vi "Actor Core.vi"(8 "error in":errorcluster, 11 "AE75TX in":refnum<class "AE75TX.lvclass">) -> (0 "error out":errorcluster, 3 "Actor out":refnum<class "Actor.lvclass">)   [LabVIEW 2015, in "AE75TX Actor.lvlib" / "AE75TX.lvclass"]
doc: "(<B>Filename</B>: Actor Framework.lvlib:Actor.lvclass:Actor Core.vi)\n\nReceives messages to the actor, reacts to them, and initiates any error handling that may shut the actor down.\n\nDescendant classes may override this VI to append parallel tasks for the actor to complete while it handles messages. Overrides use the Call Parent Method node."
uses:
  AE75TX.lvclass
  <vilib>/ActorFramework/Actor/Actor.lvclass
  Controls/PV State Selector.ctl
  AE75TX.lvclass/AE75TX.ctl
  Controls/PV Standard Value Cluster.ctl
  Controls/PV Full Data Cluster.ctl
  <vilib>/Modbus/master/Create Master Instance (TCP).vi
  <vilib>/Modbus/slave/Create Slave Instance (TCP).vi
  <vilib>/Modbus/slave/Modbus Slave.lvclass
  <vilib>/Modbus/master/Modbus Master.lvclass
panel:
  out "Deactivate":bool
  out "Activate":bool
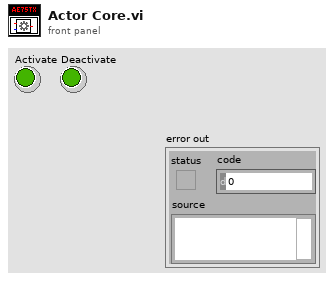
[diagram p1: front panel]
types:
  T1 = typedef "AE75TX Actor.lvlib/AE75TX.lvclass/PV State Selector.ctl" = enum16{"Init", "Read", "Error Check", "Close"}
  T2 = typedef "AE75TX Actor.lvlib/AE75TX.lvclass/PV Full Data Cluster.ctl" = cluster{"PV Standard Values":T3, "Reactive Power (kVAR)":sgl}
  T3 = typedef "AE75TX Actor.lvlib/AE75TX.lvclass/PV Standard Value Cluster.ctl" = cluster{"Va (V)":sgl, "Vb (V)":sgl, "Vc (V)":sgl, "Ia (A)":sgl, "Ib (A)":sgl, "Ic (A)":sgl, "Vdc (V)":sgl, "Idc (A)":sgl, "Frequency (Hz)":sgl, "Line Power (kW)":sgl, "Total Power (kWh)":u32, "PV Input (V)":sgl, "DC Power (kW)":sgl}
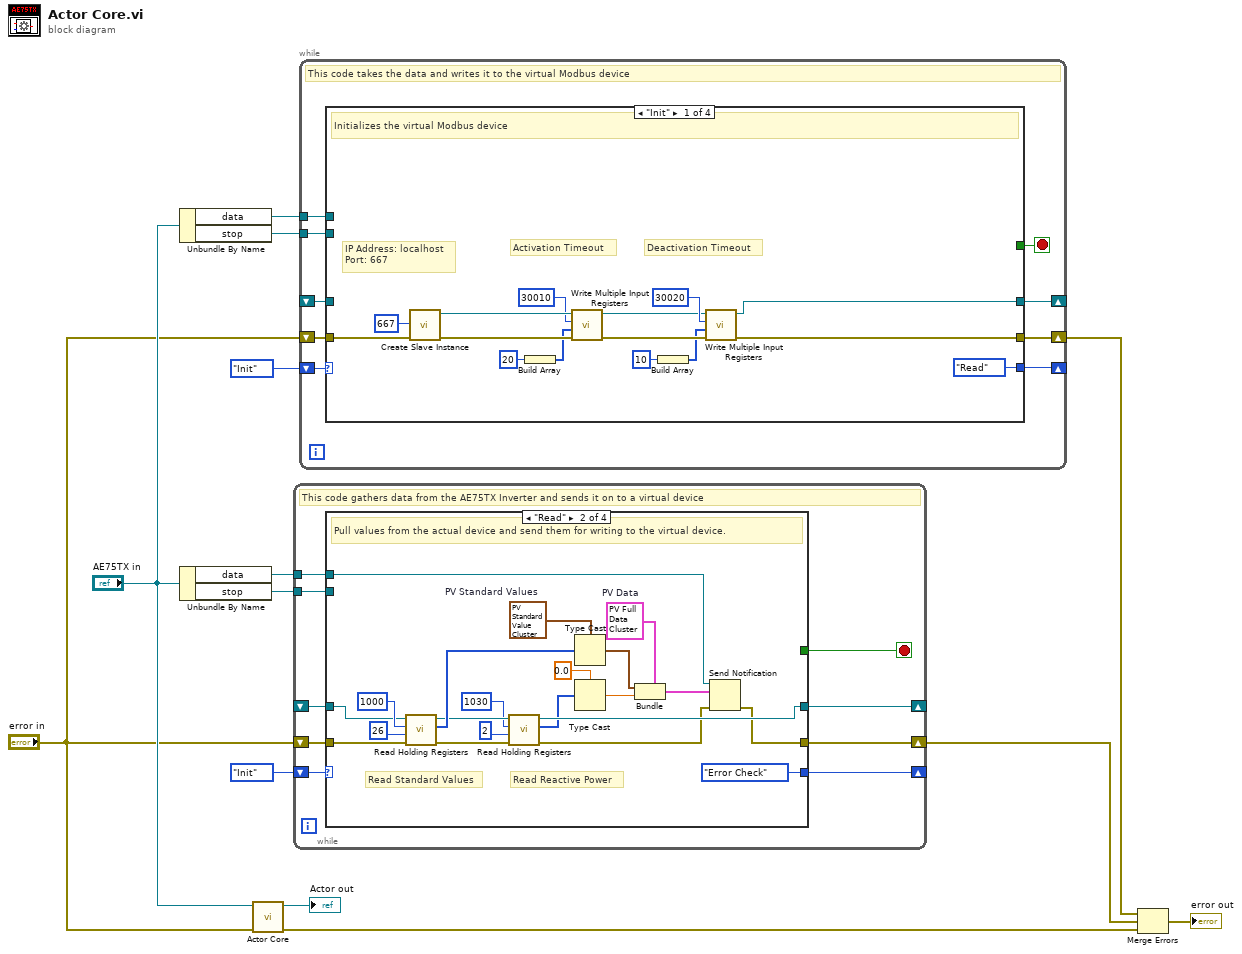
[diagram p0: block diagram]
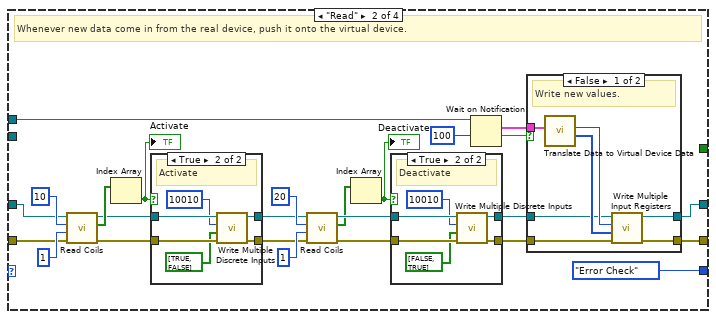
[diagram p2: hidden frame]
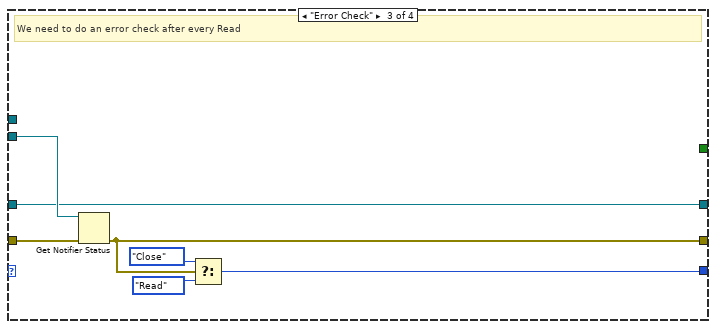
[diagram p6: hidden frame]
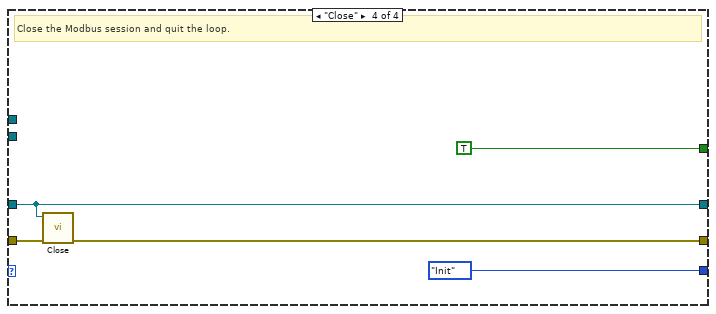
[diagram p7: hidden frame]
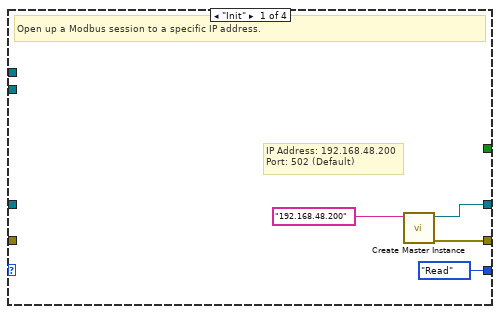
[diagram p8: hidden frame]
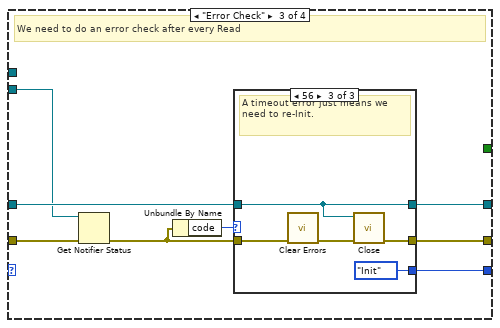
[diagram p9: hidden frame]
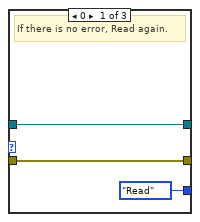
[diagram p10: hidden frame]
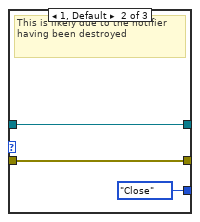
[diagram p11: hidden frame]
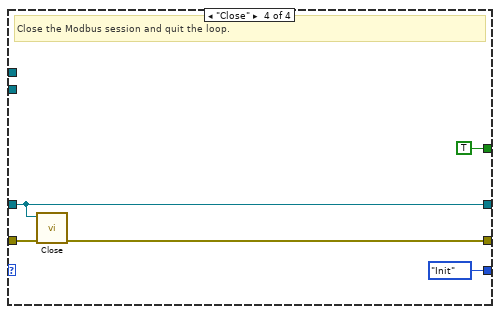
[diagram p12: hidden frame]
diagram:
  n1 = Unbundle By Name("AE75TX in") -> ("data"=w3:refnum<notifier>, "stop"=w2:refnum<notifier>)
  n2 = Unbundle By Name("AE75TX in") -> ("data"=w10:refnum<notifier>, "stop"=w9:refnum<notifier>)
  n3 = call-parent "Actor Core.vi"("error in"="error in", "Actor in"="AE75TX in") -> ("error out"=w13:errorcluster, "Actor out"=→"Actor out":refnum<class "Actor.lvclass">)  [unwired: 8 in]
  n4 = while {
    shift-right: [w20] -> _
    shift-left: PV_State_Selector."Init" -> [w22]
    shift-right: [w21] -> _
    shift-left: _ -> [w19]
    shift-right: [w17] -> w7
    shift-left: "error in" -> [w18]
    tunnel: w10 -> [w16]
    tunnel: w9 -> [w14]
    stop <- w15 stop-if-true
    # "This code gathers data from the AE75TX Inverter and sends it on to a virtual device"
    n5 = case shown="\"Read\"" w22 {
      tunnel: [w25 w37 w51 w68] -> w21
      tunnel: [w24 w27 w54 w70] -> w17
      tunnel: [PV_State_Selector."Read" PV_State_Selector."Error Check" w52 PV_State_Selector."Init"] -> w20
      tunnel: w19 -> [_ w43 w53 w68]
      tunnel: w18 -> [_ w42 w50 w71]
      tunnel: [_ _ _ TRUE ("stop")] -> w15
      tunnel: w16 -> [_ w30 _ _]
      tunnel: w14 -> [_ _ w48 _]
      frame "Init" {
        # "IP Address: 192.168.48.200\nPort: 502 (Default)"
        # "Open up a Modbus session to a specific IP address."
        n6 = call-poly <vilib>:"Create Master Instance.vi"("address"="192.168.48.200") -> ("error out"=w24:errorcluster, "TCP master instance"=w25:refnum<class "Modbus Master.lvclass">)  [unwired: 9 in]
      }
      frame "Read" {
        w31 = T2 {"PV Standard Values"={"Va (V)"=0.0, "Vb (V)"=0.0, "Vc (V)"=0.0, "Ia (A)"=0.0, "Ib (A)"=0.0, "Ic (A)"=0.0, "Vdc (V)"=0.0, "Idc (A)"=0.0, "Frequency (Hz)"=0.0, "Line Power (kW)"=0.0, "Total Power (kWh)"=0, "PV Input (V)"=0.0, "DC Power (kW)"=0.0}, "Reactive Power (kVAR)"=0.0}  # PV Data
        w46 = T3 {"Va (V)"=0.0, "Vb (V)"=0.0, "Vc (V)"=0.0, "Ia (A)"=0.0, "Ib (A)"=0.0, "Ic (A)"=0.0, "Vdc (V)"=0.0, "Idc (A)"=0.0, "Frequency (Hz)"=0.0, "Line Power (kW)"=0.0, "Total Power (kWh)"=0, "PV Input (V)"=0.0, "DC Power (kW)"=0.0}  # PV Standard Values
        # "Read Reactive Power"
        # "Read Standard Values"
        # "Pull values from the actual device and send them for writing to the virtual device."
        n7 = call-dynamic "Read Holding Registers.vi"("error in (no error)"=w42, "number of holding registers"=u16 26, "starting address"=u16 1000, "Modbus master in"=w43) -> ("error out"=w39:errorcluster, "register values"=w47:u16[], "Modbus master out"=w40:refnum<class "Modbus Master.lvclass">)  [unwired: 5 in]
        n8 = call-dynamic "Read Holding Registers.vi"("error in (no error)"=w39, "number of holding registers"=u16 2, "starting address"=u16 1030, "Modbus master in"=w40) -> ("error out"=w28:errorcluster, "register values"=w35:u16[], "Modbus master out"=w37:refnum<class "Modbus Master.lvclass">)  [unwired: 5 in]
        n9 = Type Cast(type=w46, x=w47) -> (*(type *) &x=w33:T3)
        n10 = Type Cast(type=sgl 0.0, x=w35) -> (*(type *) &x=w32:sgl)
        n11 = Bundle(cluster=w31, "PV Standard Values"=w33, "Reactive Power (kVAR)"=w32) -> (w29:T2)
        n12 = Send Notification(notification=w29, notifier=w30, error in (no error)=w28) -> (error out=w27:errorcluster)  [unwired: 1 out]
      }
      frame "Error Check" {
        # "We need to do an error check after every Read"
        n13 = Get Notifier Status(notifier=w48, error in (no error)=w50) -> (error out=w49:errorcluster)  [unwired: 4 out]
        n14 = Unbundle By Name(w49) -> ("code"=w55:i32)
        n15 = case shown="56" w55 {
          tunnel: w49 -> [w58 w59 w66]
          tunnel: [w58 w59 w64] -> w54
          tunnel: w53 -> [w57 w60 w62]
          tunnel: [PV_State_Selector."Read" PV_State_Selector."Close" PV_State_Selector."Init"] -> w52
          tunnel: [w57 w60 w62] -> w51
          frame 0 {
            # "If there is no error, Read again."
          }
          frame 1, Default {
            # "This is likely due to the notifier having been destroyed"
          }
          frame 56 {
            # "A timeout error just means we need to re-Init."
            n16 = call <vilib>:"Clear Errors.vi"("error in (no error)"=w66) -> ("error out"=w65:errorcluster)  [unwired: 5 in, 1 out]
            n17 = call-dynamic "Close.vi"("error in (no error)"=w65, "Modbus master in"=w62) -> ("error out"=w64:errorcluster)  [unwired: 9 in]
          }
        }
      }
      frame "Close" {
        # "Close the Modbus session and quit the loop."
        n18 = call-dynamic "Close.vi"("error in (no error)"=w71, "Modbus master in"=w68) -> ("error out"=w70:errorcluster)  [unwired: 9 in]
      }
    }
  }
  n19 = while {
    shift-right: [w80] -> _
    shift-left: _ -> [w76]
    shift-right: [w79] -> w1
    shift-left: "error in" -> [w75]
    tunnel: w3 -> [w74]
    tunnel: w2 -> [w73]
    shift-right: [w72] -> _
    shift-left: PV_State_Selector."Init" -> [w78]
    stop <- w77 stop-if-true
    # "This code takes the data and writes it to the virtual Modbus device"
    n20 = case shown="\"Init\"" w78 {
      tunnel: [w83 w111 w147 w153] -> w80
      tunnel: [w82 w112 w148 w154] -> w79
      tunnel: [PV_State_Selector."Read" PV_State_Selector."Error Check" w149 PV_State_Selector."Init"] -> w72
      tunnel: [_ _ _ TRUE ("stop")] -> w77
      tunnel: w76 -> [_ w110 w147 w153]
      tunnel: w75 -> [w81 w109 w146 w155]
      tunnel: w74 -> [_ w119 _ _]
      tunnel: w73 -> [_ _ w152 _]
      frame "Init" {
        # "Deactivation Timeout"
        # "Activation Timeout"
        # "IP Address: localhost\nPort: 667"
        # "Initializes the virtual Modbus device"
        n21 = call-poly <vilib>:"Create Slave Instance.vi"("error in (no error)"=w81, "port (502)"=u16 667) -> ("error out"=w92:errorcluster, "TCP slave instance"=w93:refnum<class "Modbus Slave.lvclass">)  [unwired: 8 in]
        n22 = Build Array(u16 20 ("Register")) -> (w85:u16[])
        n23 = call-dynamic "Write Multiple Input Registers.vi"("error in (no error)"=w92, "input register values"=w85, "starting address"=u16 30010, "Modbus slave in"=w93) -> ("error out"=w88:errorcluster, "Modbus slave out"=w89:refnum<class "Modbus Slave.lvclass">)  [unwired: 6 in]
        n24 = Build Array(u16 10 ("Register")) -> (w84:u16[])
        n25 = call-dynamic "Write Multiple Input Registers.vi"("error in (no error)"=w88, "input register values"=w84, "starting address"=u16 30020, "Modbus slave in"=w89) -> ("error out"=w82:errorcluster, "Modbus slave out"=w83:refnum<class "Modbus Slave.lvclass">)  [unwired: 6 in]
      }
      frame "Read" {
        # "Whenever new data come in from the real device, push it onto the virtual device."
        n26 = call-dynamic "Read Coils.vi"("error in (no error)"=w109, "number of coils"=u16 1, "starting address"=u16 10, "Modbus slave in"=w110) -> ("error out"=w114:errorcluster, "coil values"=w115:bool[], "Modbus slave out"=w113:refnum<class "Modbus Slave.lvclass">)  [unwired: 5 in]
        n27 = Index Array(array=w115) -> (element=w97:bool)  [unwired: 1 in]
        "Activate" <- w97
        n28 = case shown="True" w97 {
          tunnel: w114 -> [w138 w144]
          tunnel: w113 -> [w139 w145]
          tunnel: [w139 w141] -> w103
          tunnel: [w138 w140] -> w102
          frame False {
          }
          frame True {
            # "Activate"
            n29 = call-dynamic "Write Multiple Discrete Inputs.vi"("error in (no error)"=w144, "discrete input values"=bool[] [TRUE, FALSE], "starting address"=u16 10010, "Modbus slave in"=w145) -> ("error out"=w140:errorcluster, "Modbus slave out"=w141:refnum<class "Modbus Slave.lvclass">)  [unwired: 6 in]
          }
        }
        n30 = call-dynamic "Read Coils.vi"("error in (no error)"=w102, "number of coils"=u16 1, "starting address"=u16 20, "Modbus slave in"=w103) -> ("error out"=w107:errorcluster, "coil values"=w106:bool[], "Modbus slave out"=w108:refnum<class "Modbus Slave.lvclass">)  [unwired: 5 in]
        n31 = Index Array(array=w106) -> (element=w96:bool)  [unwired: 1 in]
        "Deactivate" <- w96
        n32 = case shown="True" w96 {
          tunnel: w107 -> [w130 w136]
          tunnel: w108 -> [w131 w137]
          tunnel: [w131 w133] -> w101
          tunnel: [w130 w132] -> w98
          frame False {
          }
          frame True {
            # "Deactivate"
            n33 = call-dynamic "Write Multiple Discrete Inputs.vi"("error in (no error)"=w136, "discrete input values"=bool[] [FALSE, TRUE], "starting address"=u16 10010, "Modbus slave in"=w137) -> ("error out"=w132:errorcluster, "Modbus slave out"=w133:refnum<class "Modbus Slave.lvclass">)  [unwired: 6 in]
          }
        }
        n34 = Wait on Notification(notifier=w119, timeout in ms (-1)=100) -> (notification=w118:T2, timed out?=w99:bool)  [unwired: 2 in, 2 out]
        n35 = case shown="False" w99 {
          tunnel: w118 -> [w122 _]
          tunnel: w98 -> [w121 w128]
          tunnel: [w125 w128] -> w112
          tunnel: [w124 w129] -> w111
          tunnel: w101 -> [w123 w129]
          frame False {
            # "Write new values."
            n36 = call "Translate Data to Virtual Device Data.vi"("PV Data"=w122) -> ("Data Array"=w126:u16[], "Address"=w127:u16)  [unwired: 9 in]
            n37 = call-dynamic "Write Multiple Input Registers.vi"("error in (no error)"=w121, "input register values"=w126, "starting address"=w127, "Modbus slave in"=w123) -> ("error out"=w125:errorcluster, "Modbus slave out"=w124:refnum<class "Modbus Slave.lvclass">)  [unwired: 6 in]
          }
          frame True {
            # "Don't write new values on a timeout."
          }
        }
      }
      frame "Error Check" {
        # "We need to do an error check after every Read"
        n38 = Get Notifier Status(notifier=w152, error in (no error)=w146) -> (error out=w148:errorcluster)  [unwired: 4 out]
        n39 = Select(t=PV_State_Selector."Close", s=w148, f=PV_State_Selector."Read") -> (s? t:f=w149:T1)
      }
      frame "Close" {
        # "Close the Modbus session and quit the loop."
        n40 = call-dynamic "Close.vi"("error in (no error)"=w155, "Modbus slave in"=w153) -> ("error out"=w154:errorcluster)  [unwired: 9 in]
      }
    }
  }
  n41 = Merge Errors(w1, w7, w13) -> (→"error out":errorcluster)
